vi "Create.vi"(8 "error in (no error)":errorcluster) -> (0 "error out":errorcluster, 3 "Barcode Detector":refnum<class "Barcode Detector.lvclass">)   [LabVIEW 2020, in "feature_detection.lvlib" / "Barcode Detector.lvclass"]
doc: "Create the Barcode Detector."
uses:
  Barcode Detector.lvclass
  Barcode Detector.lvclass/Barcode Detector.ctl
  common/common.lvlib
  common/bin/gartoolkit_fd_32-1.dll
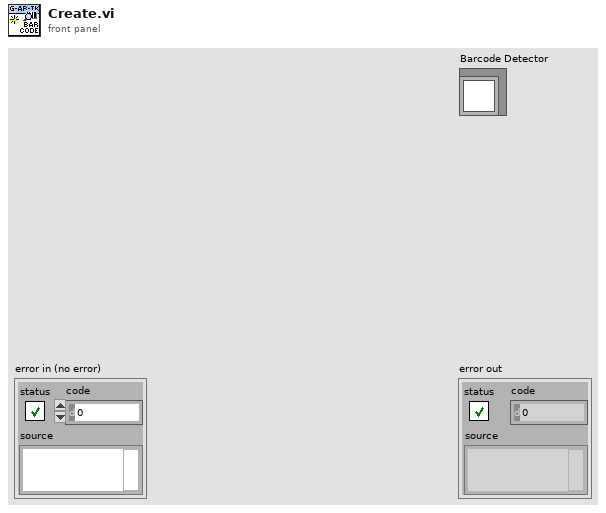
[diagram p1: front panel]
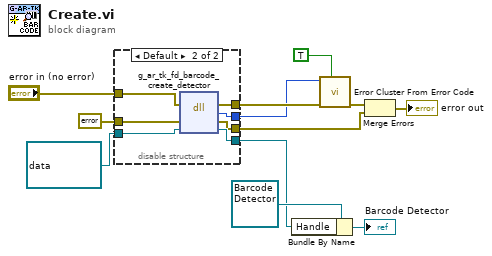
[diagram p0: block diagram]
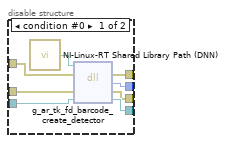
[diagram p2: hidden frame]
diagram:
  n1 = disable-structure shown="Default" {
    disable-tunnel: "error in (no error)" -> [w20 w27]
    disable-tunnel: errorcluster {"status"=FALSE, "code"=0, "source"=""} ("error constant") -> [w18 w26]
    disable-tunnel: refnum<data-value> refnum ("EDVR") -> [w17 w25]
    disable-tunnel: [w13 w24] -> w6
    disable-tunnel: [w14 w23] -> w5
    disable-tunnel: [w16 w22] -> w4
    disable-tunnel: [w15 w21] -> w1
    frame condition #0 {
      n2 = call "NI-Linux-RT Shared Library Path (DNN).vi"() -> ("Path"=w19:path)
      n3 = dll-call lib="?" fn="g_ar_tk_fd_barcode_create_detector" ("g_ar_toolkit.*.*:g_ar_tk_capture_context_create")(path in=w19, error in=w20, "error_cluster"=w18, "EDVR"=w17) -> (error out=w13:errorcluster, "return type"=w14:i32, "error_cluster"=w15:errorcluster, "EDVR"=w16:refnum<data-value>)  [unwired: 1 in, 1 out]
    }
    frame condition #1 (active) {
      n4 = dll-call lib="C:/serenial/lib/g-augmented-reality-toolkit/LabVIEW/common/bin/gartoolkit_fd_*-1.*" fn="g_ar_tk_fd_barcode_create_detector" ("g_ar_toolkit.*.*:g_ar_tk_capture_context_create")(error in=w27, "error_cluster"=w26, "EDVR"=w25) -> (error out=w24:errorcluster, "return type"=w23:i32, "error_cluster"=w21:errorcluster, "EDVR"=w22:refnum<data-value>)  [unwired: 2 in, 1 out]
    }
  }
  n5 = Bundle By Name(cluster=refnum<class "Barcode Detector.lvclass"> refnum ("Barcode Detector in"), "Handle"=w4) -> (→"Barcode Detector":refnum<class "Barcode Detector.lvclass">)
  n6 = call <vilib>:"Error Cluster From Error Code.vi"("show call chain? (False)"=TRUE, "error in (no error)"=w6, "error code (0)"=w5) -> ("error out"=w10:errorcluster)  [unwired: 6 in]
  n7 = Merge Errors(w10, w1) -> (→"error out":errorcluster)
